vi "Step Retrieve Record.vi"(8 "error in (no error)":errorcluster, 11 "Statement Refnum":T1) -> (0 "error out":errorcluster, 2 "Step":T2, 3 "Statement Refnum":T1)   [LabVIEW 2011]
uses:
  Step Record.ctl
  Summitek EXT/ODBC/SQL Controls/Statement Refnum.ctl
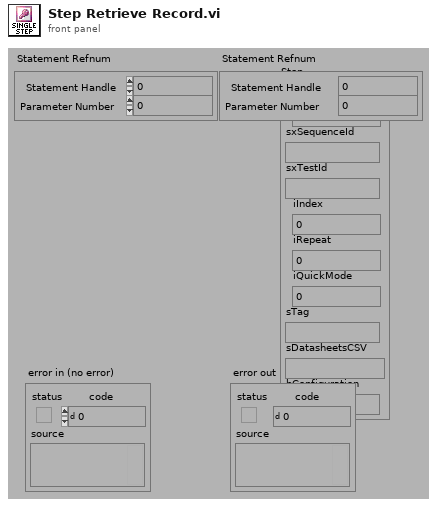
[diagram p1: front panel]
types:
  T1 = typedef "Statement Refnum.ctl" = cluster{"Statement Handle":i32, "Parameter Number":u16}
  T2 = typedef "Step Record.ctl" = cluster{"ixStep":i32, "sxSequenceId":string, "sxTestId":string, "iIndex":i32, "iRepeat":i32, "iQuickMode":i32, "sTag":string, "sDatasheetsCSV":string, "bConfiguration":string}
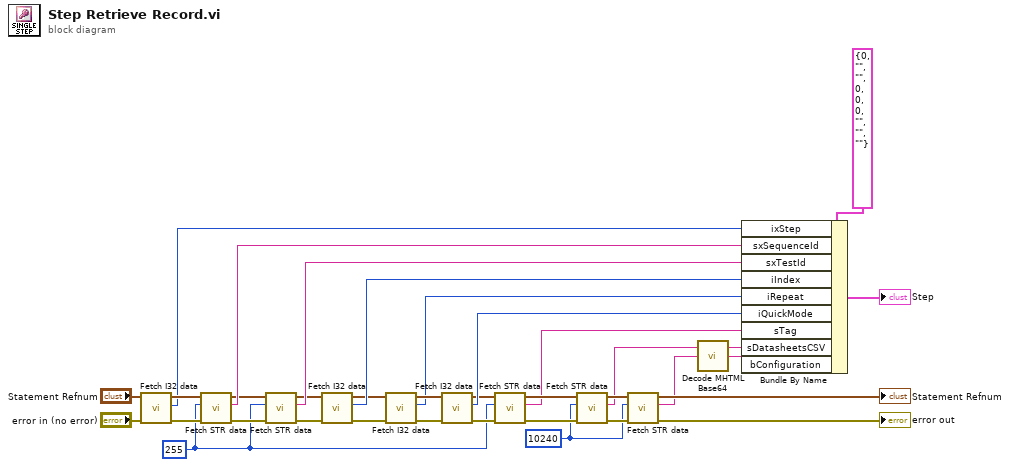
[diagram p0: block diagram]
diagram:
  w1 = 10240 ("Buffer Size")
  w9 = 255 ("Buffer Size")
  n1 = call "Fetch I32 data.vi"("error in (no error)"="error in (no error)", "Statement Refnum"="Statement Refnum") -> ("error out"=w30:errorcluster, "Data"=w28:i32, "Statement Refnum"=w32:T1)  [unwired: 3 out]
  n2 = call "Fetch STR data.vi"("error in (no error)"=w30, "Buffer Size"=w9, "Statement Refnum"=w32) -> ("error out"=w26:errorcluster, "Data"=w29:string, "Statement Refnum"=w27:T1)  [unwired: 2 out]
  n3 = call "Fetch STR data.vi"("error in (no error)"=w26, "Buffer Size"=w9, "Statement Refnum"=w27) -> ("error out"=w20:errorcluster, "Data"=w25:string, "Statement Refnum"=w21:T1)  [unwired: 2 out]
  n4 = call "Fetch I32 data.vi"("error in (no error)"=w20, "Statement Refnum"=w21) -> ("error out"=w17:errorcluster, "Data"=w19:i32, "Statement Refnum"=w18:T1)  [unwired: 3 out]
  n5 = call "Fetch I32 data.vi"("error in (no error)"=w17, "Statement Refnum"=w18) -> ("error out"=w23:errorcluster, "Data"=w16:i32, "Statement Refnum"=w24:T1)  [unwired: 3 out]
  n6 = call "Fetch I32 data.vi"("error in (no error)"=w23, "Statement Refnum"=w24) -> ("error out"=w13:errorcluster, "Data"=w15:i32, "Statement Refnum"=w14:T1)  [unwired: 3 out]
  n7 = call "Fetch STR data.vi"("error in (no error)"=w13, "Buffer Size"=w9, "Statement Refnum"=w14) -> ("error out"=w12:errorcluster, "Data"=w10:string, "Statement Refnum"=w11:T1)  [unwired: 2 out]
  n8 = call "Fetch STR data.vi"("error in (no error)"=w12, "Buffer Size"=w1, "Statement Refnum"=w11) -> ("error out"=w6:errorcluster, "Data"=w4:string, "Statement Refnum"=w8:T1)  [unwired: 2 out]
  n9 = call "Fetch STR data.vi"("error in (no error)"=w6, "Buffer Size"=w1, "Statement Refnum"=w8) -> ("error out"=→"error out":errorcluster, "Data"=w3:string, "Statement Refnum"=→"Statement Refnum":T1)  [unwired: 2 out]
  n10 = call "Decode MHTML Base64.vi"("Encoded String\n(Base64)"=w3) -> ("Decoded Binary\nString"=w2:string)  [unwired: 14 out]
  n11 = Bundle By Name(cluster=T2 {"ixStep"=0, "sxSequenceId"="", "sxTestId"="", "iIndex"=0, "iRepeat"=0, "iQuickMode"=0, "sTag"="", "sDatasheetsCSV"="", "bConfiguration"=""} ("Sequence Step Record"), "ixStep"=w28, "sxSequenceId"=w29, "sxTestId"=w25, "iIndex"=w19, "iRepeat"=w16, "iQuickMode"=w15, "sTag"=w10, "sDatasheetsCSV"=w4, "bConfiguration"=w2) -> (→"Step":T2)
